vi "NARC2017.vi"   [LabVIEW 2016, in "Moving Motor.lvrbt"]
uses:
  Moving Motor.lvrbt
  <vilib>/NXT/Block Support/NXT_InputPort.ctl
  <vilib>/NXT/Hardware/Plugins/Tetrix DC Motor/TetrixDCMotorAddress.ctl
  <vilib>/NXT/Hardware/Plugins/Tetrix 180 deg Servo/Tetrix180ServoAddress.ctl
  <vilib>/NXT/Dual Mode Library/Sensors/EV3_Color_Color.vi
  <vilib>/NXT/NXTIO Xnodes/NXTIONodeSubVIs/TETRIX IO Move Servos.vi
  <vilib>/NXT/NXTIO Xnodes/NXTIONodeSubVIs/TETRIX IO Move DC Motors.vi
  <vilib>/NXT/NXTIO Xnodes/NXTIONodeSubVIs/TETRIX IO Stop DC Motors.vi
  <vilib>/NXT/Dual Mode Library/Sensors/EV3_Ultrasonic_CM.vi
  <vilib>/NXT/NXTIO Xnodes/AddressXNode/NXTIOAddress.xnode
  <vilib>/NXT/NXTIO Xnodes/NXTIOXNode/NXTIO.xnode
  <vilib>/NXT/Subs/LVHSConnector.ctl
  <vilib>/NXT/LegoClasses/BrickReference/BrickReference.lvclass
types:
  T1 = typedef "NXT_InputPort.ctl" = u32
  T2 = typedef "LVHSConnector.ctl" = refnum<class "BrickReference.lvclass">
  T3 = typedef "Tetrix180ServoAddress.ctl" = i32
  T4 = cluster{"Tetrix180Servo":T3, "Tetrix180Servo":T3}
  T5 = typedef "TetrixDCMotorAddress.ctl" = i32
  T6 = cluster{"TetrixDCMotor":T5, "TetrixDCMotor 2":T5}
  T7 = typedef "ColorSensorColors.ctl" = enum16{"No Color", "Black", "Blue", "Green", "Yellow", "Red", "White", "Brown"}
  T8 = cluster{"Tetrix180Servo":T3, "Tetrix180Servo 2":T3}
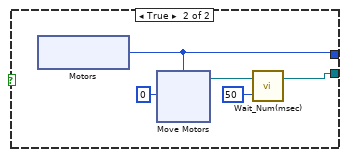
[diagram p2: hidden frame]
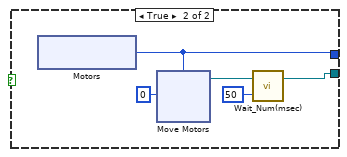
[diagram p3: hidden frame]
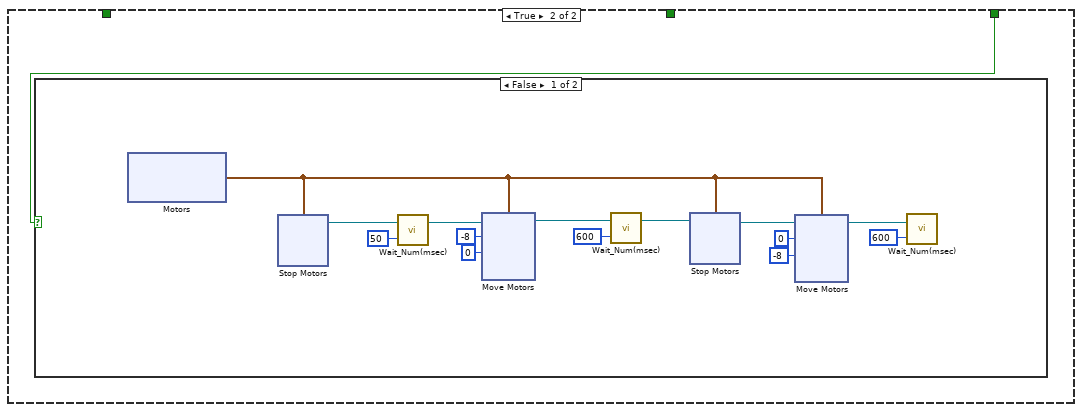
[diagram p4: hidden frame]
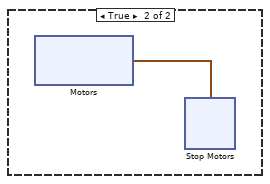
[diagram p5: hidden frame]
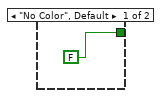
[diagram p6: hidden frame]
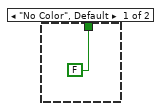
[diagram p7: hidden frame]
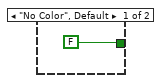
[diagram p8: hidden frame]
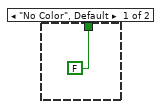
[diagram p9: hidden frame]
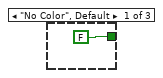
[diagram p10: hidden frame]
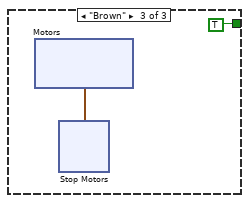
[diagram p11: hidden frame]
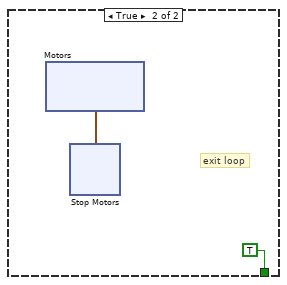
[diagram p12: hidden frame]
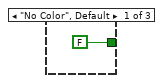
[diagram p13: hidden frame]
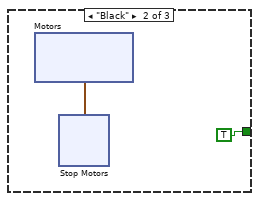
[diagram p14: hidden frame]
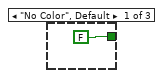
[diagram p15: hidden frame]
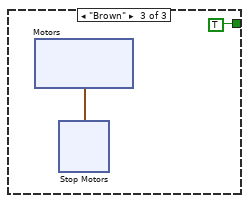
[diagram p16: hidden frame]
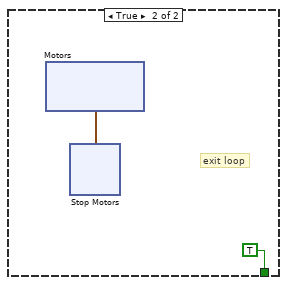
[diagram p17: hidden frame]
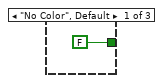
[diagram p18: hidden frame]
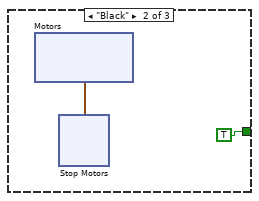
[diagram p19: hidden frame]
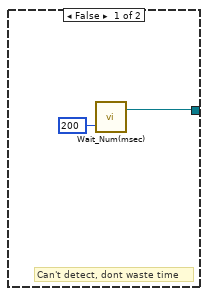
[diagram p20: hidden frame]
diagram:
  w14 = i8 10 ("Power/Speed 1")
  w69 = i8 7 ("Power/Speed 1")
  w87 = i8 -8 ("Power/Speed 1")
  w99 = i8 -8 ("Power/Speed 1")
  w109 = T1 5 items=["Port 1"=0, "Port 2"=1, "Port 3"=2, "Port 4"=3, "MidRightColor"=5] ("Port (Port 1)")
  w110 = T1 6 items=["Port 1"=0, "Port 2"=1, "Port 3"=2, "Port 4"=3, "MidLeftColor"=6] ("Port (Port 1)")
  w111 = T1 4 items=["Port 1", "Port 2", "Port 3", "Port 4", "RightColor"] ("Port (Port 1)")
  w112 = T1 7 items=["Port 1"=0, "Port 2"=1, "Port 3"=2, "Port 4"=3, "LeftColor"=7] ("Port (Port 1)")
  w121 = i8 0 ("Power/Speed 1")
  # "Turn right to enter second intersection"
  # "Go back until it detects intersection, after placing the first cube"
  # "arm and hand get into pos"
  # "move towards stacking platform, 2 seconds"
  # "drop cube"
  # "turn left to face stacking platform"
  # "Go back until it detects intersection"
  # "move forward to pickup cube"
  # "Lift cube before ultrasonic checking"
  # "turn right to enter intersection"
  # "Move backward for correction"
  # "Go to intersection slowly"
  # "Stop when it detects the first fat tape"
  # "Stop this motor instance"
  # "Let it run for 1s to pass that first thin tape"
  # "Initialize"
  n1 = call-poly <vilib>:"PolySensor.vi"("Port (Port 1)"=w111) -> ("NXT/EV3"=w108:T2)  [unwired: 2 in, 1 out]
  n2 = call-poly <vilib>:"PolySensor.vi"("NXT/EV3"=w108, "Port (Port 1)"=w109) -> ("NXT/EV3"=w107:T2)  [unwired: 1 in, 1 out]
  n3 = call-poly <vilib>:"PolySensor.vi"("NXT/EV3"=w107, "Port (Port 1)"=w110) -> ("NXT/EV3"=w106:T2)  [unwired: 1 in, 1 out]
  n4 = call-poly <vilib>:"PolySensor.vi"("NXT/EV3"=w106, "Port (Port 1)"=w112) -> ("NXT/EV3"=w105:T2)  [unwired: 1 in, 1 out]
  n5 = xnode "Motors"() -> ("Motor"=w119:T4)
  n6 = xnode "Move Servos"("Position 2"=u8 62, "Position 1"=u8 40, "Motors"=w119, "NXT/EV3"=w105) -> ("NXT/EV3"=w120:T2)
  n7 = xnode "Motors"() -> ("Motor"=w115:cluster{"TetrixDCMotor":T5, "TetrixDCMotor":T5})
  n8 = xnode "Move Motors"("Power/Speed 2"=w121, "Power/Speed 1"=w121, "Motors"=w115, "NXT/EV3"=w120) -> ("NXT/EV3"=w127:T2)
  n9 = call <vilib>:"Wait_Num(msec).vi"("Time (100 msec)"=u32 50, "NXT/EV3"=w127) -> ("NXT/EV3"=w123:T2)  [unwired: 2 in]
  n10 = xnode "Move Motors"("Power/Speed 2"=i8 12, "Power/Speed 1"=i8 14, "Motors"=w115, "NXT/EV3"=w123) -> ("NXT/EV3"=w125:T2)
  n11 = call <vilib>:"Wait_Num(msec).vi"("Time (100 msec)"=u32 3200, "NXT/EV3"=w125) -> ("NXT/EV3"=w116:T2)  [unwired: 2 in]
  n12 = xnode "Stop Motors"("Motors"=w115, "NXT/EV3"=w116) -> ("NXT/EV3"=w113:T2)
  n13 = call <vilib>:"Wait_Num(msec).vi"("Time (100 msec)"=u32 500, "NXT/EV3"=w113) -> ("NXT/EV3"=w104:T2)  [unwired: 2 in]
  n14 = while {
    tunnel: [w131] -> w88
    tunnel: w104 -> [w128]
    stop <- w132 stop-if-true
    w135 = T1 4 items=["Port 1", "Port 2", "Port 3", "Port 4", "RightColor"] ("Port (Port 1)")
    w137 = T1 7 items=["Port 1"=0, "Port 2"=1, "Port 3"=2, "Port 4"=3, "LeftColor"=7] ("Port (Port 1)")
    n15 = call-poly <vilib>:"PolySensor.vi"("Port (Port 1)"=w137) -> ("Detected Color"=w136:T7)  [unwired: 2 in, 1 out]
    n16 = call-poly <vilib>:"PolySensor.vi"("Port (Port 1)"=w135) -> ("Detected Color"=w134:T7)  [unwired: 2 in, 1 out]
    n17 = case shown="\"Black\"" w136 {
      tunnel: [FALSE TRUE TRUE] -> w130
      tunnel: w128 -> [_ w180 _]
      tunnel: w128 -> [_ _ w189]
      frame "No Color", Default {
      }
      frame "Black" {
        n18 = xnode "Motors"() -> ("Motor"=w182:cluster{"TetrixDCMotor":T5, "TetrixDCMotor":T5})
        n19 = xnode "Stop Motors"("Motors"=w182, "NXT/EV3"=w180) -> ()  [unwired: 1 out]
      }
      frame "Brown" {
        n20 = xnode "Motors"() -> ("Motor"=w190:cluster{"TetrixDCMotor":T5, "TetrixDCMotor":T5})
        n21 = xnode "Stop Motors"("Motors"=w190, "NXT/EV3"=w189) -> ()  [unwired: 1 out]
      }
    }
    n22 = case shown="\"Black\"" w134 {
      tunnel: [FALSE TRUE TRUE] -> w129
      tunnel: w128 -> [_ w139 w148]
      frame "No Color", Default {
      }
      frame "Black" {
        n23 = xnode "Motors"() -> ("Motor"=w140:cluster{"TetrixDCMotor":T5, "TetrixDCMotor":T5})
        n24 = xnode "Stop Motors"("Motors"=w140, "NXT/EV3"=w139) -> ()  [unwired: 1 out]
      }
      frame "Brown" {
        n25 = xnode "Motors"() -> ("Motor"=w149:cluster{"TetrixDCMotor":T5, "TetrixDCMotor":T5})
        n26 = xnode "Stop Motors"("Motors"=w149, "NXT/EV3"=w148) -> ()  [unwired: 1 out]
      }
    }
    n27 = Or(x=w130, y=w129) -> (x .or. y?=w133:bool)
    n28 = case shown="False" w133 {
      tunnel: [FALSE TRUE] -> w132
      tunnel: [w157 w170] -> w131
      frame False {
        w160 = i8 7 ("Power/Speed 1")
        n29 = xnode "Motors"() -> ("Motor"=w159:cluster{"TetrixDCMotor":T5, "TetrixDCMotor":T5})
        n30 = xnode "Move Motors"("Power/Speed 2"=w160, "Power/Speed 1"=w160, "Motors"=w159) -> ("NXT/EV3"=w157:T2)  [unwired: 1 in]
      }
      frame True {
        n31 = xnode "Motors"() -> ("Motor"=w171:cluster{"TetrixDCMotor":T5, "TetrixDCMotor":T5})
        n32 = xnode "Stop Motors"("Motors"=w171) -> ("NXT/EV3"=w170:T2)  [unwired: 1 in]
      }
    }
  }
  n33 = call <vilib>:"Wait_Num(msec).vi"("Time (100 msec)"=u32 1000, "NXT/EV3"=w88) -> ("NXT/EV3"=w100:T2)  [unwired: 2 in]
  n34 = xnode "Motors"() -> ("Motor"=w92:cluster{"TetrixDCMotor":T5, "TetrixDCMotor":T5})
  n35 = xnode "Move Motors"("Power/Speed 2"=w99, "Power/Speed 1"=w99, "Motors"=w92, "NXT/EV3"=w100) -> ("NXT/EV3"=w97:T2)
  n36 = call <vilib>:"Wait_Num(msec).vi"("Time (100 msec)"=u32 700, "NXT/EV3"=w97) -> ("NXT/EV3"=w93:T2)  [unwired: 2 in]
  n37 = xnode "Stop Motors"("Motors"=w92, "NXT/EV3"=w93) -> ("NXT/EV3"=w91:T2)
  n38 = xnode "Move Motors"("Power/Speed 2"=i8 0, "Power/Speed 1"=i8 16, "Motors"=w92, "NXT/EV3"=w91) -> ("NXT/EV3"=w94:T2)
  n39 = call <vilib>:"Wait_Num(msec).vi"("Time (100 msec)"=u32 1950, "NXT/EV3"=w94) -> ("NXT/EV3"=w102:T2)  [unwired: 2 in]
  n40 = xnode "Stop Motors"("Motors"=w92, "NXT/EV3"=w102) -> ("NXT/EV3"=w89:T2)
  n41 = call <vilib>:"Wait_Num(msec).vi"("Time (100 msec)"=u32 1000, "NXT/EV3"=w89) -> ("NXT/EV3"=w80:T2)  [unwired: 2 in]
  n42 = while {
    tunnel: [w198] -> w85
    tunnel: w80 -> [_]
    stop <- w201 stop-if-true
    w204 = T1 7 items=["Port 1"=0, "Port 2"=1, "Port 3"=2, "Port 4"=3, "LeftColor"=4, "RightColor"=7] ("Port (Port 1)")
    w206 = T1 4 items=["Port 1"=0, "Port 2"=1, "Port 3"=2, "Port 4"=3, "LeftColor"=4, "RightColor"=7] ("Port (Port 1)")
    n43 = call-poly <vilib>:"PolySensor.vi"("Port (Port 1)"=w206) -> ("Detected Color"=w205:T7)  [unwired: 2 in, 1 out]
    n44 = call-poly <vilib>:"PolySensor.vi"("Port (Port 1)"=w204) -> ("Detected Color"=w203:T7, "NXT/EV3"=w198:T2)  [unwired: 2 in]
    n45 = case shown="\"Brown\"" w205 {
      tunnel: [FALSE TRUE TRUE] -> w200
      frame "No Color", Default {
      }
      frame "Black" {
        n46 = xnode "Motors"() -> ("Motor"=w246:cluster{"TetrixDCMotor":T5, "TetrixDCMotor":T5})
        n47 = xnode "Stop Motors"("Motors"=w246) -> ()  [unwired: 1 in, 1 out]
      }
      frame "Brown" {
        n48 = xnode "Motors"() -> ("Motor"=w253:cluster{"TetrixDCMotor":T5, "TetrixDCMotor":T5})
        n49 = xnode "Stop Motors"("Motors"=w253) -> ()  [unwired: 1 in, 1 out]
      }
    }
    n50 = case shown="\"Black\"" w203 {
      tunnel: [FALSE TRUE TRUE] -> w199
      frame "No Color", Default {
      }
      frame "Black" {
        n51 = xnode "Motors"() -> ("Motor"=w208:cluster{"TetrixDCMotor":T5, "TetrixDCMotor":T5})
        n52 = xnode "Stop Motors"("Motors"=w208) -> ()  [unwired: 1 in, 1 out]
      }
      frame "Brown" {
        n53 = xnode "Motors"() -> ("Motor"=w216:cluster{"TetrixDCMotor":T5, "TetrixDCMotor":T5})
        n54 = xnode "Stop Motors"("Motors"=w216) -> ()  [unwired: 1 in, 1 out]
      }
    }
    n55 = Or(x=w200, y=w199) -> (x .or. y?=w202:bool)
    n56 = case shown="False" w202 {
      tunnel: [FALSE TRUE] -> w201
      frame False {
        w225 = i8 7 ("Power/Speed 1")
        # "Still following line"
        n57 = xnode "Motors"() -> ("Motor"=w224:cluster{"TetrixDCMotor":T5, "TetrixDCMotor":T5})
        n58 = xnode "Move Motors"("Power/Speed 2"=w225, "Power/Speed 1"=w225, "Motors"=w224) -> ()  [unwired: 1 in, 1 out]
      }
      frame True {
        # "exit loop"
        n59 = xnode "Motors"() -> ("Motor"=w236:cluster{"TetrixDCMotor":T5, "TetrixDCMotor":T5})
        n60 = xnode "Stop Motors"("Motors"=w236) -> ()  [unwired: 1 in, 1 out]
      }
    }
  }
  n61 = call <vilib>:"Wait_Num(msec).vi"("Time (100 msec)"=u32 200, "NXT/EV3"=w85) -> ("NXT/EV3"=w84:T2)  [unwired: 2 in]
  n62 = xnode "Motors"() -> ("Motor"=w86:cluster{"TetrixDCMotor":T5, "TetrixDCMotor":T5})
  n63 = xnode "Move Motors"("Power/Speed 2"=w87, "Power/Speed 1"=w87, "Motors"=w86, "NXT/EV3"=w84) -> ("NXT/EV3"=w81:T2)
  n64 = call <vilib>:"Wait_Num(msec).vi"("Time (100 msec)"=u32 500, "NXT/EV3"=w81) -> ("NXT/EV3"=w79:T2)  [unwired: 2 in]
  n65 = while {
    tunnel: [w261] -> w55
    tunnel: w79 -> [_]
    stop <- w262 stop-if-true
    w273 = T1 5 items=["Port 1"=0, "Port 2"=1, "Port 3"=2, "Port 4"=3, "MidRightColor"=5] ("Port (Port 1)")
    w274 = T1 6 items=["Port 1"=0, "Port 2"=1, "Port 3"=2, "Port 4"=3, "MidLeftColor"=6] ("Port (Port 1)")
    w275 = T1 4 items=["Port 1", "Port 2", "Port 3", "Port 4", "RightColor"] ("Port (Port 1)")
    w276 = T1 7 items=["Port 1"=0, "Port 2"=1, "Port 3"=2, "Port 4"=3, "LeftColor"=7] ("Port (Port 1)")
    n66 = call-poly <vilib>:"PolySensor.vi"("Port (Port 1)"=w275) -> ("Detected Color"=w269:T7, "NXT/EV3"=w261:T2)  [unwired: 2 in]
    n67 = call-poly <vilib>:"PolySensor.vi"("Port (Port 1)"=w276) -> ("Detected Color"=w272:T7)  [unwired: 2 in, 1 out]
    n68 = call-poly <vilib>:"PolySensor.vi"("Port (Port 1)"=w274) -> ("Detected Color"=w271:T7)  [unwired: 2 in, 1 out]
    n69 = call-poly <vilib>:"PolySensor.vi"("Port (Port 1)"=w273) -> ("Detected Color"=w270:T7)  [unwired: 2 in, 1 out]
    n70 = case shown="\"Black\"" w272 {
      tunnel: [FALSE TRUE] -> w265
      frame "No Color", Default {
      }
      frame "Black" {
      }
    }
    n71 = case shown="\"Black\"" w271 {
      tunnel: [FALSE TRUE] -> w268
      frame "No Color", Default {
      }
      frame "Black" {
      }
    }
    n72 = case shown="\"Black\"" w270 {
      tunnel: [FALSE TRUE] -> w267
      frame "No Color", Default {
      }
      frame "Black" {
      }
    }
    n73 = case shown="\"Black\"" w269 {
      tunnel: [FALSE TRUE] -> w264
      frame "No Color", Default {
      }
      frame "Black" {
      }
    }
    n74 = And "LC & RC"(x=w265, y=w264) -> (x .and. y?=w266:bool)
    n75 = And "MLC & MRC"(x=w268, y=w267) -> (x .and. y?=w263:bool)
    n76 = case shown="False" w266 {
      tunnel: w265 -> [w278 _]
      tunnel: w264 -> [w277 _]
      tunnel: w263 -> [_ w347]
      frame False {
        n77 = flat-sequence {
          tunnel: w278 -> [w279]
          tunnel: w277 -> [w313]
          frame #0 {
            n78 = case shown="False" w279 {
              tunnel: [w288 w300] -> w281
              tunnel: [w287 w301] -> w280
              frame False {
                n79 = xnode "Motors"() -> ("Motor"=w287:T5)
                n80 = xnode "Move Motors"("Power/Speed 1"=i8 8, "Motors"=w287) -> ("NXT/EV3"=w290:T2)  [unwired: 1 in]
                n81 = call <vilib>:"Wait_Num(msec).vi"("Time (100 msec)"=u32 80, "NXT/EV3"=w290) -> ("NXT/EV3"=w288:T2)  [unwired: 2 in]
              }
              frame True {
                n82 = xnode "Motors"() -> ("Motor"=w301:T5)
                n83 = xnode "Move Motors"("Power/Speed 1"=i8 0, "Motors"=w301) -> ("NXT/EV3"=w303:T2)  [unwired: 1 in]
                n84 = call <vilib>:"Wait_Num(msec).vi"("Time (100 msec)"=u32 50, "NXT/EV3"=w303) -> ("NXT/EV3"=w300:T2)  [unwired: 2 in]
              }
            }
            n85 = xnode "Stop Motors"("Motors"=w280, "NXT/EV3"=w281) -> ()  [unwired: 1 out]
          }
          frame #1 {
            n86 = case shown="False" w313 {
              tunnel: [w322 w334] -> w315
              tunnel: [w321 w335] -> w314
              frame False {
                n87 = xnode "Motors"() -> ("Motor"=w321:T5)
                n88 = xnode "Move Motors"("Power/Speed 1"=i8 8, "Motors"=w321) -> ("NXT/EV3"=w324:T2)  [unwired: 1 in]
                n89 = call <vilib>:"Wait_Num(msec).vi"("Time (100 msec)"=u32 80, "NXT/EV3"=w324) -> ("NXT/EV3"=w322:T2)  [unwired: 2 in]
              }
              frame True {
                n90 = xnode "Motors"() -> ("Motor"=w335:T5)
                n91 = xnode "Move Motors"("Power/Speed 1"=i8 0, "Motors"=w335) -> ("NXT/EV3"=w337:T2)  [unwired: 1 in]
                n92 = call <vilib>:"Wait_Num(msec).vi"("Time (100 msec)"=u32 50, "NXT/EV3"=w337) -> ("NXT/EV3"=w334:T2)  [unwired: 2 in]
              }
            }
            n93 = xnode "Stop Motors"("Motors"=w314, "NXT/EV3"=w315) -> ()  [unwired: 1 out]
          }
        }
      }
      frame True {
        n94 = case shown="False" w347 {
          frame False {
            n95 = xnode "Motors"() -> ("Motor"=w353:cluster{"TetrixDCMotor":T5, "TetrixDCMotor":T5})
            n96 = xnode "Stop Motors"("Motors"=w353) -> ("NXT/EV3"=w359:T2)  [unwired: 1 in]
            n97 = call <vilib>:"Wait_Num(msec).vi"("Time (100 msec)"=u32 50, "NXT/EV3"=w359) -> ("NXT/EV3"=w354:T2)  [unwired: 2 in]
            n98 = xnode "Move Motors"("Power/Speed 2"=i8 0, "Power/Speed 1"=i8 -8, "Motors"=w353, "NXT/EV3"=w354) -> ("NXT/EV3"=w356:T2)
            n99 = call <vilib>:"Wait_Num(msec).vi"("Time (100 msec)"=u32 600, "NXT/EV3"=w356) -> ("NXT/EV3"=w360:T2)  [unwired: 2 in]
            n100 = xnode "Stop Motors"("Motors"=w353, "NXT/EV3"=w360) -> ("NXT/EV3"=w350:T2)
            n101 = xnode "Move Motors"("Power/Speed 2"=i8 -8, "Power/Speed 1"=i8 0, "Motors"=w353, "NXT/EV3"=w350) -> ("NXT/EV3"=w348:T2)
            n102 = call <vilib>:"Wait_Num(msec).vi"("Time (100 msec)"=u32 600, "NXT/EV3"=w348) -> ()  [unwired: 2 in, 1 out]
          }
          frame True {
            n103 = xnode "Motors"() -> ("Motor"=w389:cluster{"TetrixDCMotor":T5, "TetrixDCMotor":T5})
            n104 = xnode "Stop Motors"("Motors"=w389) -> ()  [unwired: 1 in, 1 out]
          }
        }
      }
    }
    n105 = And "Only exit loop when all 4 sensors detect black"(x=w266, y=w263) -> (x .and. y?=w262:bool)
  }
  n106 = xnode "Motors"() -> ("Motor"=w62:T4)
  n107 = call <vilib>:"Wait_Num(msec).vi"("Time (100 msec)"=u32 200, "NXT/EV3"=w55) -> ("NXT/EV3"=w71:T2)  [unwired: 2 in]
  n108 = xnode "Move Servos"("Position 2"=u8 82, "Position 1"=u8 26, "Motors"=w62, "NXT/EV3"=w71) -> ("NXT/EV3"=w74:T2)
  n109 = xnode "Motors"() -> ("Motor"=w67:cluster{"TetrixDCMotor":T5, "TetrixDCMotor":T5})
  n110 = call-poly <vilib>:"PolyWait.vi"("Time (100 msec)"=u32 2000, "NXT/EV3"=w74) -> ("NXT/EV3"=w70:T2)  [unwired: 2 in]
  n111 = xnode "Move Motors"("Power/Speed 2"=w69, "Power/Speed 1"=w69, "Motors"=w67, "NXT/EV3"=w70) -> ("NXT/EV3"=w68:T2)
  n112 = call-poly <vilib>:"PolyWait.vi"("Time (100 msec)"=u32 1000, "NXT/EV3"=w68) -> ("NXT/EV3"=w72:T2)  [unwired: 2 in]
  n113 = xnode "Stop Motors"("Motors"=w67, "NXT/EV3"=w72) -> ("NXT/EV3"=w66:T2)
  n114 = call-poly <vilib>:"PolyWait.vi"("Time (100 msec)"=u32 200, "NXT/EV3"=w66) -> ("NXT/EV3"=w63:T2)  [unwired: 2 in]
  n115 = xnode "Move Servos"("Position 2"=u8 0, "Position 1"=u8 90, "Motors"=w62, "NXT/EV3"=w63) -> ("NXT/EV3"=w60:T2)
  n116 = call-poly <vilib>:"PolyWait.vi"("Time (100 msec)"=u32 3000, "NXT/EV3"=w60) -> ("NXT/EV3"=w58:T2)  [unwired: 2 in]
  n117 = call-poly <vilib>:"PolySensor.vi"("NXT/EV3"=w58) -> ("Centimeters"=w57:sgl)  [unwired: 2 in, 1 out]
  n118 = Less?(x=w57, y=sgl 7.0) -> (x < y?=w52:bool)
  n119 = case shown="False" w52 {
    tunnel: [w404 w481] -> w53
    frame False {
      w408 = T1 0 items=["Port 1", "Port 2", "Port 3", "Port 4"] ("Port (Port 1)")
      w412 = i8 7 ("Power/Speed 1")
      w432 = i8 -10 ("Power/Speed 1")
      # "Added error handling cube isn't picked up"
      # "move forward to pickup cube"
      # "Life cube before ultrasonic checking"
      n120 = xnode "Motors"() -> ("Motor"=w411:cluster{"TetrixDCMotor":T5, "TetrixDCMotor":T5})
      n121 = xnode "Move Motors"("Power/Speed 2"=w432, "Power/Speed 1"=w432, "Motors"=w411) -> ("NXT/EV3"=w431:T2)  [unwired: 1 in]
      n122 = call <vilib>:"Wait_Num(msec).vi"("Time (100 msec)"=u32 500, "NXT/EV3"=w431) -> ("NXT/EV3"=w429:T2)  [unwired: 2 in]
      n123 = xnode "Motors"() -> ("Motor"=w410:T4)
      n124 = xnode "Stop Motors"("Motors"=w411, "NXT/EV3"=w429) -> ("NXT/EV3"=w416:T2)
      n125 = xnode "Move Servos"("Position 2"=u8 82, "Position 1"=u8 26, "Motors"=w410, "NXT/EV3"=w416) -> ("NXT/EV3"=w414:T2)
      n126 = call-poly <vilib>:"PolyWait.vi"("Time (100 msec)"=u32 2000, "NXT/EV3"=w414) -> ("NXT/EV3"=w413:T2)  [unwired: 2 in]
      n127 = xnode "Move Motors"("Power/Speed 2"=w412, "Power/Speed 1"=w412, "Motors"=w411, "NXT/EV3"=w413) -> ("NXT/EV3"=w426:T2)
      n128 = call-poly <vilib>:"PolyWait.vi"("Time (100 msec)"=u32 1500, "NXT/EV3"=w426) -> ("NXT/EV3"=w427:T2)  [unwired: 2 in]
      n129 = xnode "Stop Motors"("Motors"=w411, "NXT/EV3"=w427) -> ("NXT/EV3"=w425:T2)
      n130 = call-poly <vilib>:"PolyWait.vi"("Time (100 msec)"=u32 200, "NXT/EV3"=w425) -> ("NXT/EV3"=w422:T2)  [unwired: 2 in]
      n131 = xnode "Move Servos"("Position 2"=u8 0, "Position 1"=u8 90, "Motors"=w410, "NXT/EV3"=w422) -> ("NXT/EV3"=w421:T2)
      n132 = call-poly <vilib>:"PolyWait.vi"("Time (100 msec)"=u32 3000, "NXT/EV3"=w421) -> ("NXT/EV3"=w419:T2)  [unwired: 2 in]
      n133 = call-poly <vilib>:"PolySensor.vi"("NXT/EV3"=w419, "Port (Port 1)"=w408) -> ("Centimeters"=w406:sgl)  [unwired: 1 in, 1 out]
      n134 = Less?(x=w406, y=sgl 7.0) -> (x < y?=w405:bool)
      n135 = case shown="True" w405 {
        tunnel: [w433 w435] -> w404
        frame False {
          # "Can't detect, dont waste time"
          n136 = call <vilib>:"Wait_Num(msec).vi"("Time (100 msec)"=u32 200) -> ("NXT/EV3"=w433:T2)  [unwired: 3 in]
        }
        frame True {
          n137 = call <vilib>:"Wait_Num(msec).vi"("Time (100 msec)"=u32 200) -> ("NXT/EV3"=w435:T2)  [unwired: 3 in]
        }
      }
    }
    frame True {
      n138 = call <vilib>:"Wait_Num(msec).vi"("Time (100 msec)"=u32 200) -> ("NXT/EV3"=w481:T2)  [unwired: 3 in]
    }
  }
  n139 = call-poly <vilib>:"PolyWait.vi"("Time (100 msec)"=u32 500, "NXT/EV3"=w53) -> ("NXT/EV3"=w51:T2)  [unwired: 2 in]
  n140 = while {
    tunnel: [w483] -> w49
    tunnel: w51 -> [_]
    stop <- w486 stop-if-true
    w489 = T1 7 items=["Port 1"=0, "Port 2"=1, "Port 3"=2, "Port 4"=3, "LeftColor"=4, "RightColor"=7] ("Port (Port 1)")
    w491 = T1 4 items=["Port 1"=0, "Port 2"=1, "Port 3"=2, "Port 4"=3, "LeftColor"=4, "RightColor"=7] ("Port (Port 1)")
    n141 = call-poly <vilib>:"PolySensor.vi"("Port (Port 1)"=w491) -> ("Detected Color"=w490:T7)  [unwired: 2 in, 1 out]
    n142 = call-poly <vilib>:"PolySensor.vi"("Port (Port 1)"=w489) -> ("Detected Color"=w488:T7, "NXT/EV3"=w483:T2)  [unwired: 2 in]
    n143 = case shown="\"Brown\"" w490 {
      tunnel: [FALSE TRUE TRUE] -> w485
      frame "No Color", Default {
      }
      frame "Black" {
        n144 = xnode "Motors"() -> ("Motor"=w531:cluster{"TetrixDCMotor":T5, "TetrixDCMotor":T5})
        n145 = xnode "Stop Motors"("Motors"=w531) -> ()  [unwired: 1 in, 1 out]
      }
      frame "Brown" {
        n146 = xnode "Motors"() -> ("Motor"=w538:cluster{"TetrixDCMotor":T5, "TetrixDCMotor":T5})
        n147 = xnode "Stop Motors"("Motors"=w538) -> ()  [unwired: 1 in, 1 out]
      }
    }
    n148 = case shown="\"Black\"" w488 {
      tunnel: [FALSE TRUE TRUE] -> w484
      frame "No Color", Default {
      }
      frame "Black" {
        n149 = xnode "Motors"() -> ("Motor"=w493:cluster{"TetrixDCMotor":T5, "TetrixDCMotor":T5})
        n150 = xnode "Stop Motors"("Motors"=w493) -> ()  [unwired: 1 in, 1 out]
      }
      frame "Brown" {
        n151 = xnode "Motors"() -> ("Motor"=w501:cluster{"TetrixDCMotor":T5, "TetrixDCMotor":T5})
        n152 = xnode "Stop Motors"("Motors"=w501) -> ()  [unwired: 1 in, 1 out]
      }
    }
    n153 = Or(x=w485, y=w484) -> (x .or. y?=w487:bool)
    n154 = case shown="False" w487 {
      tunnel: [FALSE TRUE] -> w486
      frame False {
        w510 = i8 -7 ("Power/Speed 1")
        # "Still following line"
        n155 = xnode "Motors"() -> ("Motor"=w509:cluster{"TetrixDCMotor":T5, "TetrixDCMotor":T5})
        n156 = xnode "Move Motors"("Power/Speed 2"=w510, "Power/Speed 1"=w510, "Motors"=w509) -> ()  [unwired: 1 in, 1 out]
      }
      frame True {
        # "exit loop"
        n157 = xnode "Motors"() -> ("Motor"=w521:cluster{"TetrixDCMotor":T5, "TetrixDCMotor":T5})
        n158 = xnode "Stop Motors"("Motors"=w521) -> ()  [unwired: 1 in, 1 out]
      }
    }
  }
  n159 = call-poly <vilib>:"PolyWait.vi"("Time (100 msec)"=u32 500, "NXT/EV3"=w49) -> ("NXT/EV3"=w43:T2)  [unwired: 2 in]
  n160 = xnode "Motors"() -> ("Motor"=w19:cluster{"TetrixDCMotor":T5, "TetrixDCMotor":T5})
  n161 = xnode "Move Motors"("Power/Speed 2"=i8 17, "Power/Speed 1"=i8 -16, "Motors"=w19, "NXT/EV3"=w43) -> ("NXT/EV3"=w45:T2)
  n162 = call <vilib>:"Wait_Num(msec).vi"("Time (100 msec)"=u32 900, "NXT/EV3"=w45) -> ("NXT/EV3"=w44:T2)  [unwired: 2 in]
  n163 = xnode "Stop Motors"("Motors"=w19, "NXT/EV3"=w44) -> ("NXT/EV3"=w18:T2)
  n164 = xnode "Motors"() -> ("Motor"=w25:T4)
  n165 = call-poly <vilib>:"PolyWait.vi"("Time (100 msec)"=u32 500, "NXT/EV3"=w18) -> ("NXT/EV3"=w16:T2)  [unwired: 2 in]
  n166 = xnode "Move Servos"("Position 2"=u8 62, "Position 1"=u8 60, "Motors"=w25, "NXT/EV3"=w16) -> ("NXT/EV3"=w39:T2)
  n167 = call <vilib>:"Wait_Num(msec).vi"("Time (100 msec)"=u32 500, "NXT/EV3"=w39) -> ("NXT/EV3"=w36:T2)  [unwired: 2 in]
  n168 = xnode "Move Servos"("Position 2"=u8 115, "Position 1"=u8 110, "Motors"=w25, "NXT/EV3"=w36) -> ("NXT/EV3"=w33:T2)
  n169 = xnode "Motors"() -> ("Motor"=w27:cluster{"TetrixDCMotor":T5, "TetrixDCMotor":T5})
  n170 = call <vilib>:"Wait_Num(msec).vi"("Time (100 msec)"=u32 2000, "NXT/EV3"=w33) -> ("NXT/EV3"=w32:T2)  [unwired: 2 in]
  n171 = xnode "Move Motors"("Power/Speed 2"=i8 10, "Power/Speed 1"=i8 10, "Motors"=w27, "NXT/EV3"=w32) -> ("NXT/EV3"=w29:T2)
  n172 = call <vilib>:"Wait_Num(msec).vi"("Time (100 msec)"=u32 2500, "NXT/EV3"=w29) -> ("NXT/EV3"=w28:T2)  [unwired: 2 in]
  n173 = xnode "Stop Motors"("Motors"=w27, "NXT/EV3"=w28) -> ("NXT/EV3"=w23:T2)
  n174 = xnode "Move Servos"("Position 2"=u8 110, "Position 1"=u8 80, "Motors"=w25, "NXT/EV3"=w23) -> ("NXT/EV3"=w21:T2)
  n175 = call <vilib>:"Wait_Num(msec).vi"("Time (100 msec)"=u32 1000, "NXT/EV3"=w21) -> ("NXT/EV3"=w15:T2)  [unwired: 2 in]
  n176 = while {
    tunnel: [w546] -> w2
    tunnel: w15 -> [_]
    stop <- w549 stop-if-true
    w552 = T1 7 items=["Port 1"=0, "Port 2"=1, "Port 3"=2, "Port 4"=3, "LeftColor"=4, "RightColor"=7] ("Port (Port 1)")
    w554 = T1 4 items=["Port 1"=0, "Port 2"=1, "Port 3"=2, "Port 4"=3, "LeftColor"=4, "RightColor"=7] ("Port (Port 1)")
    n177 = call-poly <vilib>:"PolySensor.vi"("Port (Port 1)"=w554) -> ("Detected Color"=w553:T7)  [unwired: 2 in, 1 out]
    n178 = call-poly <vilib>:"PolySensor.vi"("Port (Port 1)"=w552) -> ("Detected Color"=w551:T7, "NXT/EV3"=w546:T2)  [unwired: 2 in]
    n179 = case shown="\"Brown\"" w553 {
      tunnel: [FALSE TRUE TRUE] -> w548
      frame "No Color", Default {
      }
      frame "Black" {
        n180 = xnode "Motors"() -> ("Motor"=w594:cluster{"TetrixDCMotor":T5, "TetrixDCMotor":T5})
        n181 = xnode "Stop Motors"("Motors"=w594) -> ()  [unwired: 1 in, 1 out]
      }
      frame "Brown" {
        n182 = xnode "Motors"() -> ("Motor"=w601:cluster{"TetrixDCMotor":T5, "TetrixDCMotor":T5})
        n183 = xnode "Stop Motors"("Motors"=w601) -> ()  [unwired: 1 in, 1 out]
      }
    }
    n184 = case shown="\"Black\"" w551 {
      tunnel: [FALSE TRUE TRUE] -> w547
      frame "No Color", Default {
      }
      frame "Black" {
        n185 = xnode "Motors"() -> ("Motor"=w556:cluster{"TetrixDCMotor":T5, "TetrixDCMotor":T5})
        n186 = xnode "Stop Motors"("Motors"=w556) -> ()  [unwired: 1 in, 1 out]
      }
      frame "Brown" {
        n187 = xnode "Motors"() -> ("Motor"=w564:cluster{"TetrixDCMotor":T5, "TetrixDCMotor":T5})
        n188 = xnode "Stop Motors"("Motors"=w564) -> ()  [unwired: 1 in, 1 out]
      }
    }
    n189 = Or(x=w548, y=w547) -> (x .or. y?=w550:bool)
    n190 = case shown="False" w550 {
      tunnel: [FALSE TRUE] -> w549
      frame False {
        w573 = i8 -7 ("Power/Speed 1")
        # "Still following line"
        n191 = xnode "Motors"() -> ("Motor"=w572:cluster{"TetrixDCMotor":T5, "TetrixDCMotor":T5})
        n192 = xnode "Move Motors"("Power/Speed 2"=w573, "Power/Speed 1"=w573, "Motors"=w572) -> ()  [unwired: 1 in, 1 out]
      }
      frame True {
        # "exit loop"
        n193 = xnode "Motors"() -> ("Motor"=w584:cluster{"TetrixDCMotor":T5, "TetrixDCMotor":T5})
        n194 = xnode "Stop Motors"("Motors"=w584) -> ()  [unwired: 1 in, 1 out]
      }
    }
  }
  n195 = call <vilib>:"Wait_Num(msec).vi"("Time (100 msec)"=u32 100, "NXT/EV3"=w2) -> ("NXT/EV3"=w12:T2)  [unwired: 2 in]
  n196 = xnode "Motors"() -> ("Motor"=w4:cluster{"TetrixDCMotor":T5, "TetrixDCMotor":T5})
  n197 = xnode "Move Motors"("Power/Speed 2"=w14, "Power/Speed 1"=w14, "Motors"=w4, "NXT/EV3"=w12) -> ("NXT/EV3"=w10:T2)
  n198 = call <vilib>:"Wait_Num(msec).vi"("Time (100 msec)"=u32 1300, "NXT/EV3"=w10) -> ("NXT/EV3"=w8:T2)  [unwired: 2 in]
  n199 = xnode "Move Motors"("Power/Speed 2"=i8 -16, "Power/Speed 1"=i8 0, "Motors"=w4, "NXT/EV3"=w8) -> ("NXT/EV3"=w6:T2)
  n200 = call <vilib>:"Wait_Num(msec).vi"("Time (100 msec)"=u32 1850, "NXT/EV3"=w6) -> ("NXT/EV3"=w5:T2)  [unwired: 2 in]
  n201 = xnode "Stop Motors"("Motors"=w4, "NXT/EV3"=w5) -> ("NXT/EV3"=w1:T2)
  n202 = while {
    tunnel: [w609] -> _
    tunnel: w1 -> [_]
    stop <- w610 stop-if-true
    w621 = T1 5 items=["Port 1"=0, "Port 2"=1, "Port 3"=2, "Port 4"=3, "MidRightColor"=5] ("Port (Port 1)")
    w622 = T1 6 items=["Port 1"=0, "Port 2"=1, "Port 3"=2, "Port 4"=3, "MidLeftColor"=6] ("Port (Port 1)")
    w623 = T1 4 items=["Port 1", "Port 2", "Port 3", "Port 4", "RightColor"] ("Port (Port 1)")
    w624 = T1 7 items=["Port 1"=0, "Port 2"=1, "Port 3"=2, "Port 4"=3, "LeftColor"=7] ("Port (Port 1)")
    n203 = call-poly <vilib>:"PolySensor.vi"("Port (Port 1)"=w623) -> ("Detected Color"=w617:T7, "NXT/EV3"=w609:T2)  [unwired: 2 in]
    n204 = call-poly <vilib>:"PolySensor.vi"("Port (Port 1)"=w624) -> ("Detected Color"=w620:T7)  [unwired: 2 in, 1 out]
    n205 = call-poly <vilib>:"PolySensor.vi"("Port (Port 1)"=w622) -> ("Detected Color"=w619:T7)  [unwired: 2 in, 1 out]
    n206 = call-poly <vilib>:"PolySensor.vi"("Port (Port 1)"=w621) -> ("Detected Color"=w618:T7)  [unwired: 2 in, 1 out]
    n207 = case shown="\"Black\"" w620 {
      tunnel: [FALSE TRUE] -> w613
      frame "No Color", Default {
      }
      frame "Black" {
      }
    }
    n208 = case shown="\"Black\"" w619 {
      tunnel: [FALSE TRUE] -> w616
      frame "No Color", Default {
      }
      frame "Black" {
      }
    }
    n209 = case shown="\"Black\"" w618 {
      tunnel: [FALSE TRUE] -> w615
      frame "No Color", Default {
      }
      frame "Black" {
      }
    }
    n210 = case shown="\"Black\"" w617 {
      tunnel: [FALSE TRUE] -> w612
      frame "No Color", Default {
      }
      frame "Black" {
      }
    }
    n211 = And "LC & RC"(x=w613, y=w612) -> (x .and. y?=w614:bool)
    n212 = And "MLC & MRC"(x=w616, y=w615) -> (x .and. y?=w611:bool)
    n213 = case shown="False" w614 {
      tunnel: w613 -> [w626 _]
      tunnel: w612 -> [w625 _]
      tunnel: w611 -> [_ w695]
      frame False {
        n214 = flat-sequence {
          tunnel: w626 -> [w627]
          tunnel: w625 -> [w661]
          frame #0 {
            n215 = case shown="False" w627 {
              tunnel: [w636 w648] -> w629
              tunnel: [w635 w649] -> w628
              frame False {
                n216 = xnode "Motors"() -> ("Motor"=w635:T5)
                n217 = xnode "Move Motors"("Power/Speed 1"=i8 8, "Motors"=w635) -> ("NXT/EV3"=w638:T2)  [unwired: 1 in]
                n218 = call <vilib>:"Wait_Num(msec).vi"("Time (100 msec)"=u32 80, "NXT/EV3"=w638) -> ("NXT/EV3"=w636:T2)  [unwired: 2 in]
              }
              frame True {
                n219 = xnode "Motors"() -> ("Motor"=w649:T5)
                n220 = xnode "Move Motors"("Power/Speed 1"=i8 0, "Motors"=w649) -> ("NXT/EV3"=w651:T2)  [unwired: 1 in]
                n221 = call <vilib>:"Wait_Num(msec).vi"("Time (100 msec)"=u32 50, "NXT/EV3"=w651) -> ("NXT/EV3"=w648:T2)  [unwired: 2 in]
              }
            }
            n222 = xnode "Stop Motors"("Motors"=w628, "NXT/EV3"=w629) -> ()  [unwired: 1 out]
          }
          frame #1 {
            n223 = case shown="False" w661 {
              tunnel: [w670 w682] -> w663
              tunnel: [w669 w683] -> w662
              frame False {
                n224 = xnode "Motors"() -> ("Motor"=w669:T5)
                n225 = xnode "Move Motors"("Power/Speed 1"=i8 8, "Motors"=w669) -> ("NXT/EV3"=w672:T2)  [unwired: 1 in]
                n226 = call <vilib>:"Wait_Num(msec).vi"("Time (100 msec)"=u32 80, "NXT/EV3"=w672) -> ("NXT/EV3"=w670:T2)  [unwired: 2 in]
              }
              frame True {
                n227 = xnode "Motors"() -> ("Motor"=w683:T5)
                n228 = xnode "Move Motors"("Power/Speed 1"=i8 0, "Motors"=w683) -> ("NXT/EV3"=w685:T2)  [unwired: 1 in]
                n229 = call <vilib>:"Wait_Num(msec).vi"("Time (100 msec)"=u32 50, "NXT/EV3"=w685) -> ("NXT/EV3"=w682:T2)  [unwired: 2 in]
              }
            }
            n230 = xnode "Stop Motors"("Motors"=w662, "NXT/EV3"=w663) -> ()  [unwired: 1 out]
          }
        }
      }
      frame True {
        n231 = case shown="False" w695 {
          frame False {
            n232 = xnode "Motors"() -> ("Motor"=w701:cluster{"TetrixDCMotor":T5, "TetrixDCMotor":T5})
            n233 = xnode "Stop Motors"("Motors"=w701) -> ("NXT/EV3"=w707:T2)  [unwired: 1 in]
            n234 = call <vilib>:"Wait_Num(msec).vi"("Time (100 msec)"=u32 50, "NXT/EV3"=w707) -> ("NXT/EV3"=w702:T2)  [unwired: 2 in]
            n235 = xnode "Move Motors"("Power/Speed 2"=i8 0, "Power/Speed 1"=i8 -8, "Motors"=w701, "NXT/EV3"=w702) -> ("NXT/EV3"=w704:T2)
            n236 = call <vilib>:"Wait_Num(msec).vi"("Time (100 msec)"=u32 600, "NXT/EV3"=w704) -> ("NXT/EV3"=w708:T2)  [unwired: 2 in]
            n237 = xnode "Stop Motors"("Motors"=w701, "NXT/EV3"=w708) -> ("NXT/EV3"=w698:T2)
            n238 = xnode "Move Motors"("Power/Speed 2"=i8 -8, "Power/Speed 1"=i8 0, "Motors"=w701, "NXT/EV3"=w698) -> ("NXT/EV3"=w696:T2)
            n239 = call <vilib>:"Wait_Num(msec).vi"("Time (100 msec)"=u32 600, "NXT/EV3"=w696) -> ()  [unwired: 2 in, 1 out]
          }
          frame True {
            n240 = xnode "Motors"() -> ("Motor"=w737:cluster{"TetrixDCMotor":T5, "TetrixDCMotor":T5})
            n241 = xnode "Stop Motors"("Motors"=w737) -> ()  [unwired: 1 in, 1 out]
          }
        }
      }
    }
    n242 = And "Only exit loop when all 4 sensors detect black"(x=w614, y=w611) -> (x .and. y?=w610:bool)
  }
